vi "FPGA1483_8tap8_GPU.vi"() -> ()   [LabVIEW 2013]
doc: "This is the FPGA VI for the 10-Tap 8-Bit Camera with DRAM example. This example demonstrates how to acquire images from a 10-tap, 8-bit, extended configuration, Camera Link camera and transfer the images to the host. This example supports area scan and line scan cameras for both continuous and finite acquisitions.\n\nThis example also demonstrates the use of DRAM as a frame buffer for very high speed acquisitions. Data packing and flow-control are also employed to maximize use of the available DRAM and FIFOs in terms of both memory space and performance.\n\nAdditionally, the example demonstrates the serial server, which allows third-party camera configuration utilities to communicate with the camera using the Camera Link serial interface while this VI is running."
uses:
  <vilib>/Platform/TimedLoop/XDataNode/timing_clust.ctl
  <vilib>/Platform/TimedLoop/XDataNode/nitl_modes.ctl
  <vilib>/Platform/TimedLoop/XDataNode/wakeup.ctl
  <vilib>/rvi/eio/common/nirviEmuTemplateMethod_errors.vi
  <vilib>/rvi/Emulation/niFpgaSctlEmulationGetInTimedLoop.vi
  <vilib>/rvi/Emulation/niFpgaEmulationReportErrorSimple.vi
  <vilib>/rvi/Emulation/niFpgaGetClockAttributes.vi
  <vilib>/rvi/Emulation/niFpgaCriticalErrorInLSC.vi
  Common/CL Data to Pixels/8 Tap 8-Bit.vi
  <vilib>/rvi/interface/RandomDataEmulation/nirviRandomDataFPGAFIFO.vi
  <vilib>/rvi/interface/RandomDataEmulation/niFpgaRandomDataHandleErrors.vi
  <vilib>/rvi/Emulation/niFpgaProcessEmulError.vi
  <vilib>/Platform/TimedLoop/XDataNode/XDataNode.xnode
  <vilib>/eio/EIONode/EIONode.xnode
  <vilib>/rvi/DataTransferAndStorage/Container/XNode/niFpgaContainer.xnode
  <vilib>/rvi/interface/RandomDataEmulation/nirviRandomDataFpgaReadWriteTemplate.vi
  <vilib>/Platform/TimedLoop/XDataNode/XDNodeRunTimeDep.lvlib
panel:
  in  "Tab Control":T1(tab)=enum."IMAQ GPU Profile"
  out "Platform":enum8{"FlexRIO", "cRIO", "RSeries"}(ring)
  out "FPGAVIversion":u8[](array[numeric])=[1, 1]
  out "InitDone":bool
  out "InsertedIOModule ID":u32=278099145
  out "RIOAdapterCorrect":bool
  out "Fref":u32=100000000
  out "DevTemp":i16=147
  out "DevProfile":u8=3
  in  "DAQStartStop":bool
  in  "DebugMode":bool
  out "DevQualityStatus":u8
  out "DMATtoGPUNCh":u16[](array[numeric])=[1]
  out "DMATtoGPUBlockNWords":u16[](array[numeric])=[8192]
  in  "DMATtoGPUEnable0":bool
  in  "DMATtoGPUSamplingRate0":u16
  out "DMATtoGPUOverflows":u16
  out "DMATtoGPUSampleSize":u8[](array[numeric])=[1]
  out "DMATtoGPUFrameType":u8[](array[numeric])
  in  "SpareHigh":bool=TRUE caption="CL Config.Spare Active High"
  in  "FVALHigh":bool=TRUE caption="CL Config.FVAL Active High"
  in  "LVALHigh":bool=TRUE caption="CL Config.LVAL Active High"
  in  "DVALHigh":bool=TRUE caption="CL Config.DVAL Active High"
  in  "LineScan":bool caption="CL Config.Line Scan"
  in  "SignalMapping":u8 caption="CL Config.Signal Mapping"
  in  "Configuration":u8=2 caption="CL Config.Configuration"
  in  "ControlEnable":bool=TRUE caption="IO Module\\CL Control Enable"
  in  "uartReceive":bool caption="UART.Receive"
  out "uartRxByte":u8 caption="UART.Rx Data" format="%02x"
  out "uartTxReady":bool caption="UART.Tx Ready"
  out "uartOverrunError":bool caption="UART.Overrun Error"
  out "uartFramingError":bool caption="UART.Framing Error"
  out "uartBreakIndicator":bool caption="UART.Break Indicator"
  out "uartRxReady":bool caption="auxDI1"
  in  "uartByteMode":bool=TRUE caption="UART.Byte Mode"
  in  "uartSetBaudRate":bool caption="UART.Set Baud Rate"
  in  "uartTransmit":bool caption="UART.Transmit"
  in  "uartBaudRate":u8=1 caption="UART.Baud Rate"
  in  "uartTxByte":u8=1 caption="DataBytetoTx" format="%x"
  out "DI0":bool
  out "DI1":bool
  in  "auxAO0":i32
  out "auxAI1":i32
  out "SGNo":u8
  in  "DO0":bool
  in  "DO1":bool
  out "auxAI0":i32
  out "Acq Status.Lines Per Frame":u32
  out "Acq Status.Frames Acq'd":u32
  out "Acq Status.Clocks Per Line":u32
  out "Acq Status.Acq In Progress":bool
  in  "Acq Control.Ignore DVAL":bool
  in  "Acq Control.Frames To Acq":u32
  in  "Acq Control.Line Scan Height":u32
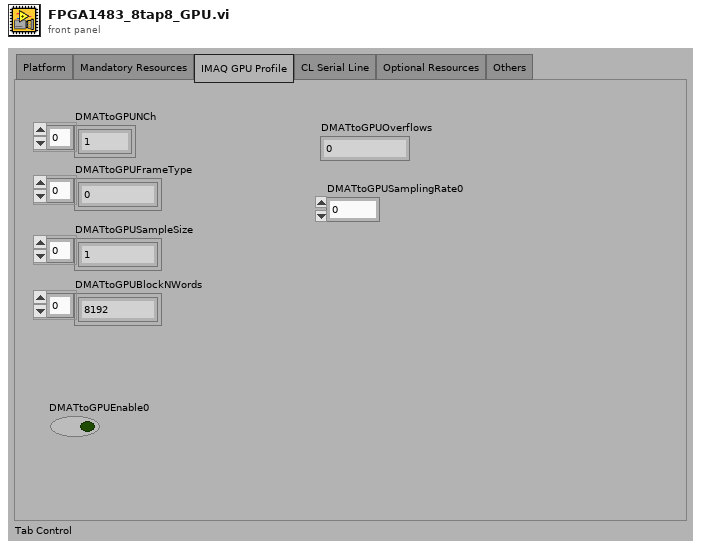
[diagram p1: front panel]
types:
  T1 = enum32{"Platform", "Mandatory Resources", "IMAQ GPU Profile", "CL Serial Line", "Optional Resources", "Others"}
  T2 = typedef "XDNodeRunTimeDep.lvlib/timing_clust.ctl" = cluster{"Expected End [f-1]":u64, "Actual End [f-1]":u64, "Finished Late? [f-1]":bool, "Expected End [i-1]":u64, "Actual End [i-1]":u64, "Finished Late? [i-1]":bool, "Expected Start [i]":u64, "Actual Start [i]":u64, "Expected Start [f]":u64, "Actual Start [f]":u64, "Source Name":string, "Structure Name":string, "Period":i64, "Deadline":i64, "Offset":i64, "Start":i64, "Priority":i32, "Timeout":i32, "Mode":T3, "Wakeup Reason":T4, "Error":errorcluster, "Source Type":string, "Secondary Source Type":string, "Global End Time":u64, "Global Start Time":u64, "Frame Duration":u64, "Iteration Duration":u64, "Assigned CPU":i32, "I/O Scan Engine Mode":u32}
  T3 = typedef "XDNodeRunTimeDep.lvlib/nitl_modes.ctl" = enum32{"No Change", "Process missed periods, maintain original phase", "Discard missed periods, maintain original phase", "Process missed periods, ignore original phase", "Discard missed periods, ignore original phase"}
  T4 = typedef "XDNodeRunTimeDep.lvlib/wakeup.ctl" = enum32{"Normal", "Aborted", "Asynchronous wakeup", "Timing source error", "Timed loop error", "Timeout"}
  T5 = cluster{"Enables Valid":bool, "Frame Valid":bool, "Line Valid":bool, "Data Valid":bool}
  T6 = enum8{"Standard", "Basler 10-tap", "Vosskühler 10-tap"}
  T7 = cluster{"Pixel 0":u8, "Pixel 1":u8, "Pixel 2":u8, "Pixel 3":u8, "Pixel 4":u8, "Pixel 5":u8, "Pixel 6":u8, "Pixel 7":u8}
  T8 = cluster{"Tx Data":u8[], "Transmit":bool, "Receive":bool, "Byte Mode":bool, "Set Baud Rate":bool, "Baud Rate":u8}
  T9 = cluster{"Rx Data":u8, "Turn Off Transmit":bool, "Turn Off Receive":bool, "Turn Off Set Baud Rate":bool, "Tx Ready":bool, "Rx Ready":bool, "Break Indicator":bool, "Framing Error":bool, "Overrun Error":bool}
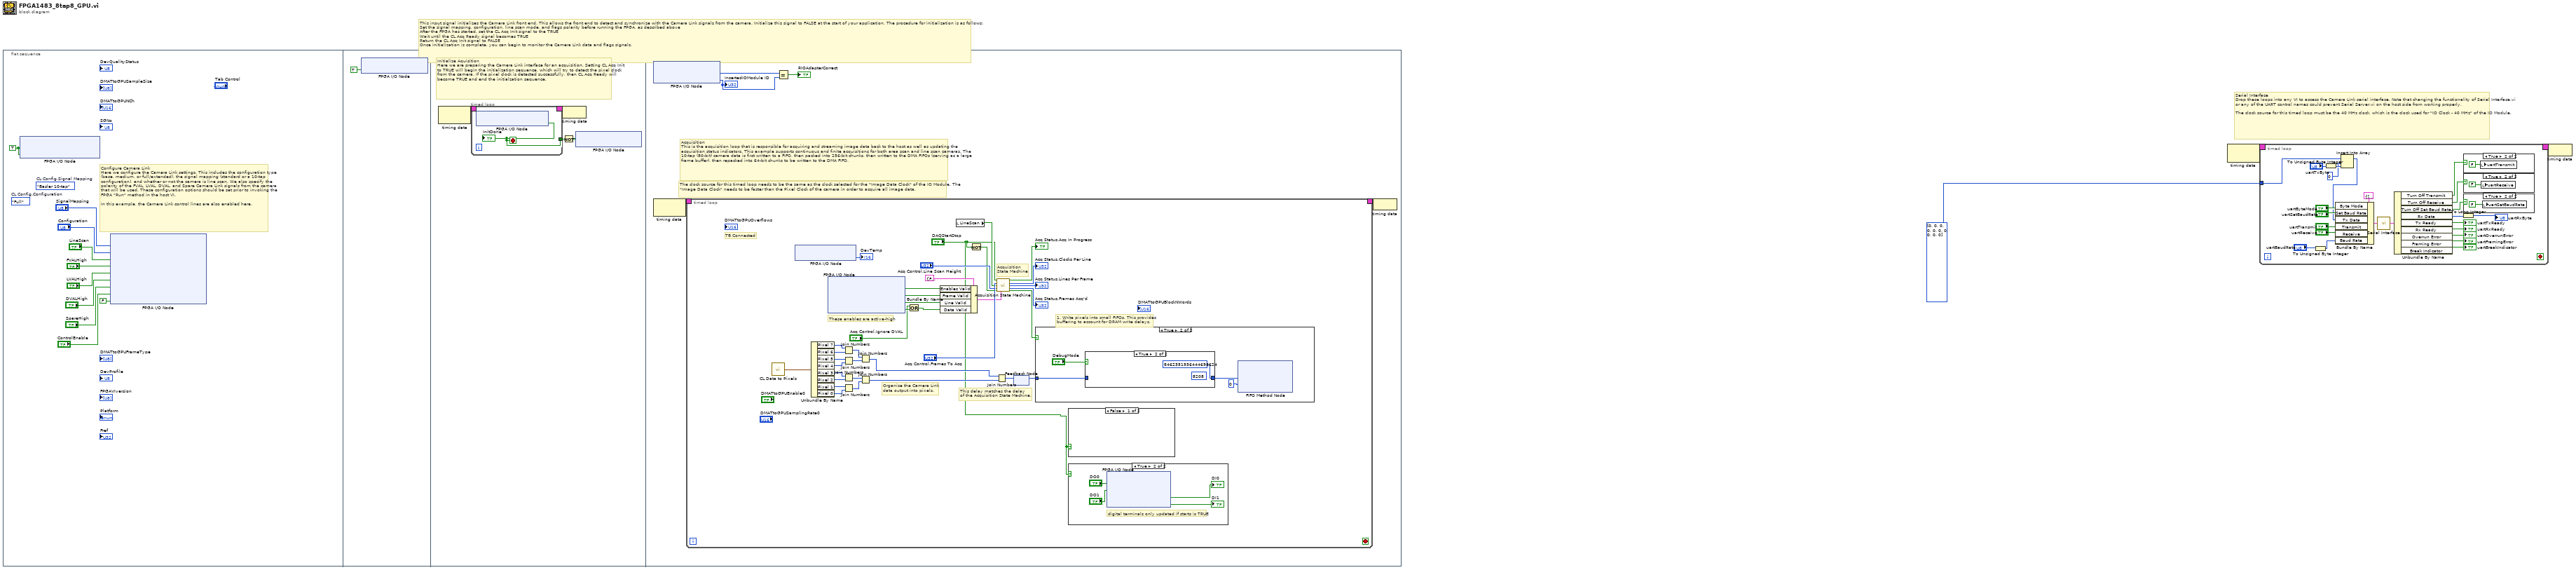
[diagram p0: block diagram]
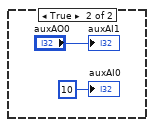
[diagram p5: hidden frame]
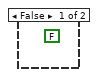
[diagram p7: hidden frame]
diagram:
  # "This input signal initializes the Camera Link front end. This allows the front end to detect and synchronize with the Camera Link signals from the camera. Initialize this signal to FALSE at the start of your application. The procedure for initialization is as follows: \nSet the signal mapping, configuration, line scan mode, and flags polarity before running the FPGA, as described above \nAfter the FPGA has started, set the CL Acq Init signal to the TRUE \nWait until the CL Acq Ready signal becomes TRUE \nReturn the CL Acq Init signal to FALSE \nOnce initialization is complete, you can begin to monitor the Camera Link data and flags signals."
  # "Serial Interface\nDrop these loops into any VI to access the Camera Link serial interface. Note that changing the functionality of Serial Interface.vi or any of the UART control names could prevent Serial Server.vi on the host side from working properly.\n\nThe clock source for this timed loop must be the 40 MHz clock, which is the clock used for \"IO Clock - 40 MHz\" of the IO Module."
  n1 = flat-sequence {
    frame #0 {
      w4 = TRUE ("IO Module\\TTL Out Enable 0")
      (unwired) T6."Basler 10-tap"  # CL Config.Signal Mapping
      (unwired) enum8{"Base", "Medium", "Full"}."Full"  # CL Config.Configuration
      # "Configure Camera Link\nHere we configure the Camera Link settings. This includes the configuration type (base, medium, or full/extended), the signal mapping (standard or a 10-tap configuration), and whether or not the camera is line scan. We also specify the polarity of the FVAL, LVAL, DVAL, and Spare Camera Link signals from the camera that will be used. These configuration options should be set prior to invoking the FPGA \"Run\" method in the host VI.\n\nIn this example, the Camera Link control lines are also enabled here."
      n2 = xnode "FPGA I/O Node"("IO Module\\TTL Out Enable 0"=w4, "IO Module\\TTL Out Enable 1"=w4) -> ()  [unwired: 2 in, 2 out]
      n3 = xnode "FPGA I/O Node"("IO Module\\CL Set Signal Mapping"="SignalMapping", "IO Module\\CL Set Configuration"="Configuration", "IO Module\\CL Set Line Scan"="LineScan", "IO Module\\CL Set FVAL Active High"="FVALHigh", "IO Module\\CL Set LVAL Active High"="LVALHigh", "IO Module\\CL Set DVAL Active High"="DVALHigh", "IO Module\\CL Set Spare Active High"="SpareHigh", "IO Module\\CL Control Enable"="ControlEnable", "IO Module\\CL Acq Init"=FALSE ("IO Module\\CL Acq Init")) -> ()  [unwired: 9 in, 9 out]
    }
    frame #1 {
      n4 = xnode "FPGA I/O Node"("IO Module\\CL Acq Init"=TRUE) -> ()  [unwired: 1 in, 1 out]
    }
    frame #2 {
      # "Initialize Aquisition\nHere we are preparing the Camera Link interface for an acquisition. Setting CL Acq Init to TRUE will begin the initialization sequence, which will try to detect the pixel clock from the camera. If the pixel clock is detected successfully, then CL Acq Ready will become TRUE and end the initialzation sequence."
      n5 = node-c288() -> (w18:T2)  [unwired: 1 out]
      n6 = timed-loop {
        timing: w18 -> [_]
        timing-out: [_] -> w17
        tunnel: [w19] -> w16
        stop <- w19 stop-if-true
        n7 = xnode "FPGA I/O Node"() -> ("IO Module\\CL Acq Ready"=w19:bool)  [unwired: 1 in, 1 out]
        "InitDone" <- w19
      }
      n8 = node-c288(w17) -> ()
      n9 = Not(x=w16) -> (.not. x?=w15:bool)
      n10 = xnode "FPGA I/O Node"("IO Module\\CL Acq Init"=w15) -> ()  [unwired: 1 in, 1 out]
    }
    frame #3 {
      # "The clock source for this timed loop needs to be the same as the clock selected for the \"Image Data Clock\" of the IO Module. The \"Image Data Clock\" needs to be faster than the Pixel Clock of the camera in order to acquire all image data."
      # "Acquisition\nThis is the acquisition loop that is responsible for acquiring and streaming image data back to the host as well as updating the acquisition status indicators. This example supports continuous and finite acquisitions for both area scan and line scan cameras. The 10-tap (80-bit) camera data is first written to a FIFO, then packed into 256-bit chunks, then written to the DMA FIFOs (serving as a large frame buffer), then repacked into 64-bit chunks to be written to the DMA FIFO."
      n11 = xnode "FPGA I/O Node"() -> ("Expected IO Module ID"=w26:u32, "Inserted IO Module ID"=w25:u32)  [unwired: 2 in, 2 out]
      "InsertedIOModule ID" <- w25
      n12 = node-c288() -> (w28:T2)  [unwired: 1 in]
      n13 = timed-loop {
        timing: w28 -> [_]
        timing-out: [_] -> w27
        stop <- _ stop-if-true
        # "TB Connected"
        # "1. Write pixels into small FIFOs. This provides\nbuffering to account for DRAM write delays."
        # "Organize the Camera Link\ndata output into pixels."
        # "These enables are active-high"
        # "This delay matches the delay\nof the Acquisition State Machine."
        # "Acquisition\nState Machine"
        n14 = call-poly "CL Data to Pixels.vi"() -> ("Pixels"=w64:T7)  [unwired: 1 in]
        n15 = xnode "FPGA I/O Node"() -> ("Device Temperature"=→"DevTemp":i16)  [unwired: 1 in, 1 out]
        n16 = Unbundle By Name(w64) -> ("Pixel 7"=w46:u8, "Pixel 6"=w45:u8, "Pixel 5"=w44:u8, "Pixel 4"=w43:u8, "Pixel 3"=w42:u8, "Pixel 2"=w41:u8, "Pixel 1"=w40:u8, "Pixel 0"=w39:u8)
        n17 = xnode "FPGA I/O Node"() -> ("IO Module\\CL Output Valid"=w56:bool, "IO Module\\CL Frame Valid"=w55:bool, "IO Module\\CL Line Valid"=w54:bool, "IO Module\\CL Data Valid"=w51:bool)  [unwired: 4 in, 4 out]
        n18 = Join Numbers(hi=w46, lo=w45) -> ((hi.lo)=w37:u16)
        n19 = Join Numbers(hi=w44, lo=w43) -> ((hi.lo)=w36:u16)
        n20 = Join Numbers(hi=w42, lo=w41) -> ((hi.lo)=w35:u16)
        n21 = Join Numbers(hi=w40, lo=w39) -> ((hi.lo)=w38:u16)
        n22 = Join Numbers(hi=w37, lo=w36) -> ((hi.lo)=w34:u32)
        n23 = Join Numbers(hi=w35, lo=w38) -> ((hi.lo)=w33:u32)
        n24 = Or(x="Acq Control.Ignore DVAL", y=w51) -> (x .or. y?=w50:bool)
        n25 = Bundle By Name(cluster=T5 {"Enables Valid"=FALSE, "Frame Valid"=FALSE, "Line Valid"=FALSE, "Data Valid"=FALSE} ("Enables"), "Enables Valid"=w56, "Frame Valid"=w55, "Line Valid"=w54, "Data Valid"=w50) -> (w53:T5)
        n26 = local read "LineScan"() -> (w48:bool)
        n27 = Not(x="DAQStartStop") -> (.not. x?=w31:bool)
        n28 = Join Numbers(hi=w34, lo=w33) -> ((hi.lo)=w32:u64)
        n29 = call "Acquisition State Machine.vi"("Acquire"="DAQStartStop", "Frames to Acquire"="Acq Control.Frames To Acq", "Line Scan"=w48, "Line Scan Height"="Acq Control.Line Scan Height", "Cancel Acq"=w31, "Enables"=w53) -> ("Acq In Progress"=→"Acq Status.Acq In Progress":bool, "Num Clocks Per Line"=→"Acq Status.Clocks Per Line":u32, "Num Lines Per Frame"=→"Acq Status.Lines Per Frame":u32, "Num Frames Acq'd"=→"Acq Status.Frames Acq'd":u32, "Capture Cycle"=w62:bool)  [unwired: 4 in, 1 out]
        n30 = feedback-in #1(w32) -> ()
        n31 = feedback #1() -> (w63:u64)  [unwired: 1 in]
        n32 = case shown="True" w62 {
          tunnel: w63 -> [_ w72]
          frame False {
            (unwired) FALSE ("Timed Out?")
          }
          frame True {
            n33 = case shown="True" "DebugMode" {
              tunnel: w72 -> [w75 _]
              tunnel: [w75 u64 8462351936444698624] -> w71
              frame False {
              }
              frame True {
                (unwired) u16 8208
              }
            }
            n34 = xnode ("FIFO Method Node")("Element"=w71, "Timeout"=0) -> ()  [unwired: 1 in, 2 out]
          }
        }
        n35 = case shown="False" "DAQStartStop" {
          frame False {
          }
          frame True {
            "auxAI0" <- i16 10 ("auxAI0")
            "auxAI1" <- "auxAO0"
          }
        }
        n36 = case shown="True" "DAQStartStop" {
          frame False {
          }
          frame True {
            # "digital terminals only updated if starts is TRUE"
            n37 = xnode "FPGA I/O Node"("IO Module\\TTL Out 0"="DO0", "IO Module\\TTL Out 1"="DO1") -> ("IO Module\\TTL In 2"=→"DI0":bool, "IO Module\\TTL In 3"=→"DI1":bool)  [unwired: 4 in, 4 out]
          }
        }
      }
      n38 = Equal?(x=w26, y=w25) -> (x = y?=→"RIOAdapterCorrect":bool)
      n39 = node-c288(w27) -> ()
    }
  }
  n40 = node-c288() -> (w3:T2)  [unwired: 1 out]
  n41 = timed-loop {
    timing: w3 -> [_]
    timing-out: [_] -> w2
    tunnel: u8[] [0, 0, 0, 0, 0, 0, 0, 0, 0, 0] -> [w86]
    stop <- _ stop-if-true
    n42 = To Unsigned Byte Integer(number="uartBaudRate") -> (unsigned 8bit integer=w83:u8)
    n43 = To Unsigned Byte Integer(number="uartTxByte") -> (unsigned 8bit integer=w89:u8)
    n44 = Insert Into Array(array=w86, index=0, new element=w89) -> (w85:u8[])
    n45 = Bundle By Name(cluster=T8 {"Tx Data"=[0, 0, 0, 0, 0, 0, 0, 0, 0, 0], "Transmit"=FALSE, "Receive"=FALSE, "Byte Mode"=TRUE, "Set Baud Rate"=FALSE, "Baud Rate"=0} ("UART Inputs"), "Byte Mode"="uartByteMode", "Set Baud Rate"="uartSetBaudRate", "Tx Data"=w85, "Transmit"="uartTransmit", "Receive"="uartReceive", "Baud Rate"=w83) -> (w90:T8)
    n46 = call "Serial Interface.vi"("UART Inputs"=w90) -> ("UART Outputs"=w100:T9)
    n47 = Unbundle By Name(w100) -> ("Turn Off Transmit"=w93:bool, "Turn Off Receive"=w94:bool, "Turn Off Set Baud Rate"=w92:bool, "Rx Data"=w81:u8, "Tx Ready"=→"uartTxReady":bool, "Rx Ready"=→"uartRxReady":bool, "Overrun Error"=→"uartOverrunError":bool, "Framing Error"=→"uartFramingError":bool, "Break Indicator"=→"uartBreakIndicator":bool)
    n48 = To Long Integer(number=w81) -> (32bit integer=→"uartRxByte":i32)
    n49 = case shown="True" w93 {
      frame False {
      }
      frame True {
        n50 = local write "uartTransmit"(FALSE ("UART.Transmit")) -> ()
      }
    }
    n51 = case shown="True" w94 {
      frame False {
      }
      frame True {
        n52 = local write "uartReceive"(FALSE ("UART.Receive")) -> ()
      }
    }
    n53 = case shown="True" w92 {
      frame False {
      }
      frame True {
        n54 = local write "uartSetBaudRate"(FALSE ("UART.Receive")) -> ()
      }
    }
  }
  n55 = node-c288(w2) -> ()
